vi "XML_Read_Modbus_Items.vi"(8 "error in (no error)":errorcluster, 11 ".NET Refnum in":refnum<k24>) -> (0 "error out":errorcluster, 2 "Array":T1[](array[typedef]), 3 ".NET Refnum out":refnum<k24>)   [LabVIEW 2014, in "XML_Deserializer.lvlib"]
uses:
  XML_Deserializer.lvlib
  C:/Users/vruault.AMER/Desktop/Source code/XML Deserializer/.NET Files/bin/Debug/Modbus_CD_XML_Deserializer.dll
  .NET Files/bin/Debug/Modbus_CD_XML_Deserializer.dll
  Controls/Modbus_Items.ctl
  Controls/Modbus_Item_Type.ctl
  Shared/Modbus Shared.lvlib
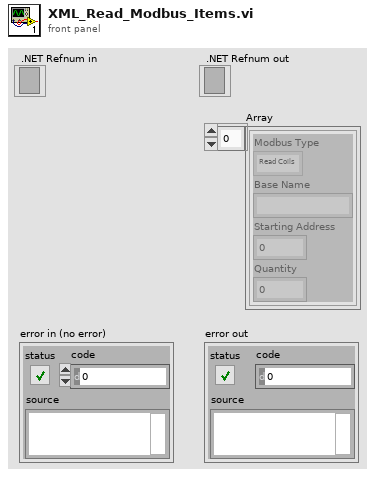
[diagram p1: front panel]
types:
  T1 = typedef "Modbus Shared.lvlib/Modbus_Items.ctl" = cluster{"Modbus Type":T2, "Base Name":string, "Starting Address":u16, "Quantity":u16}
  T2 = typedef "Modbus Shared.lvlib/Modbus_Item_Type.ctl" = enum16{"Read Coils", "Read Discrete Inputs", "Read Holding Registers", "Read Input Registers", "Write Multiple Coils", "Write Multiple Holding Registers", "Write Single Coil", "Write Single Holding Register", "Write Multiple Discrete Inputs", "Write Multiple Input Registers"}
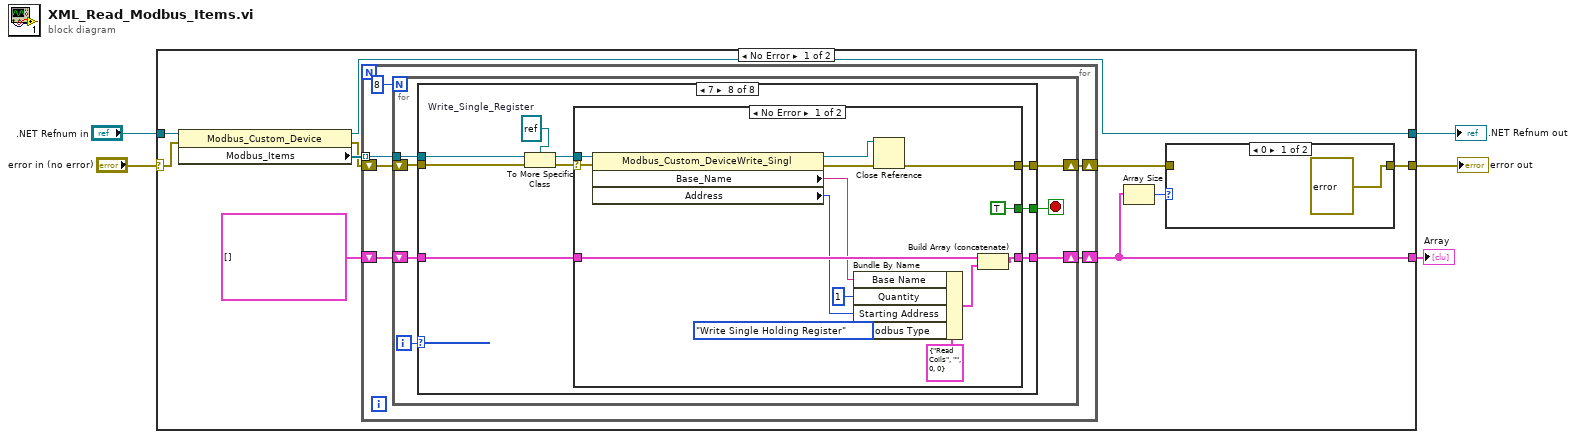
[diagram p0: block diagram]
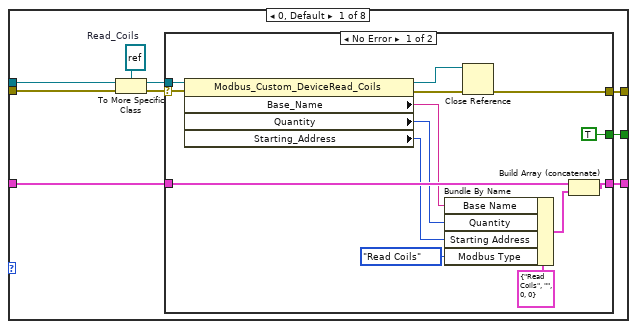
[diagram p3: hidden frame]
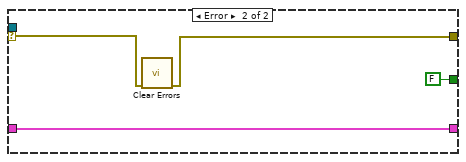
[diagram p4: hidden frame]
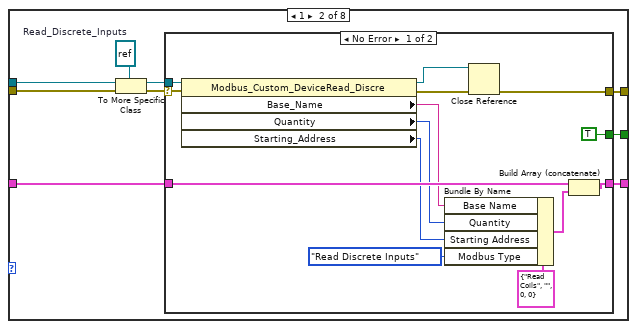
[diagram p5: hidden frame]
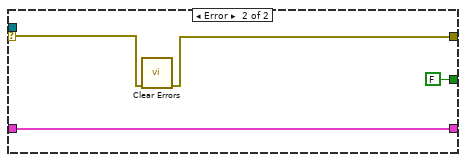
[diagram p6: hidden frame]
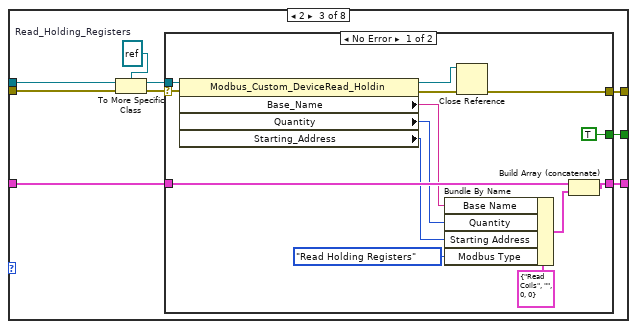
[diagram p7: hidden frame]
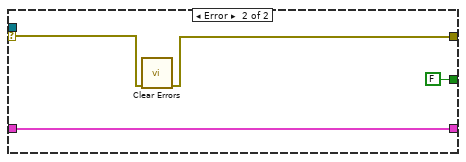
[diagram p8: hidden frame]
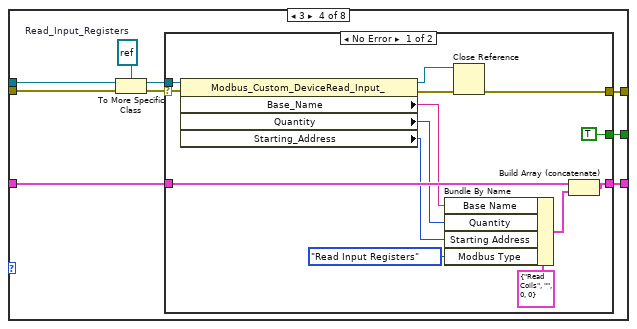
[diagram p9: hidden frame]
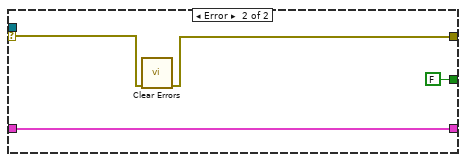
[diagram p10: hidden frame]
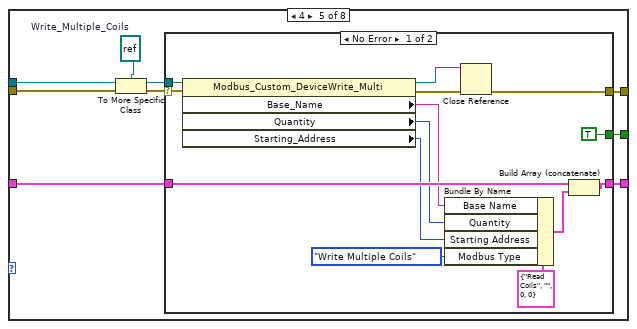
[diagram p11: hidden frame]
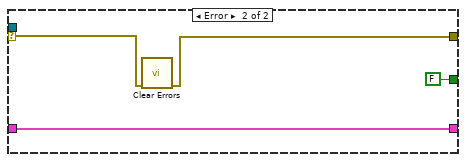
[diagram p12: hidden frame]
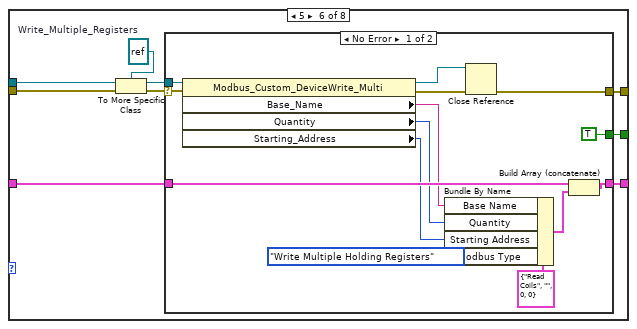
[diagram p13: hidden frame]
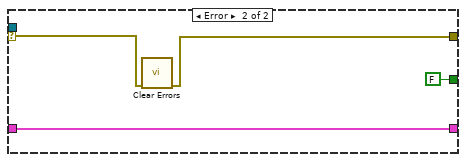
[diagram p14: hidden frame]
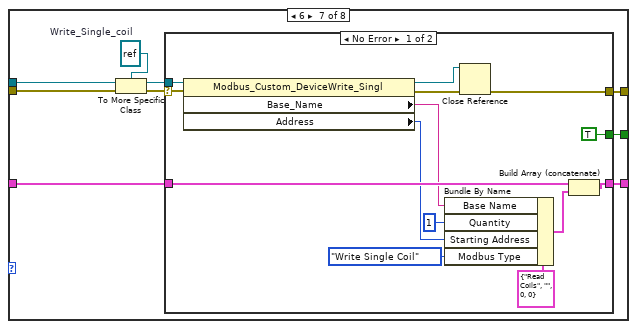
[diagram p15: hidden frame]
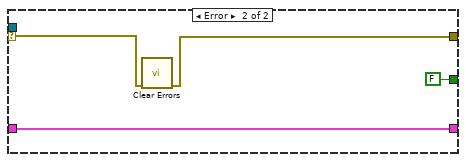
[diagram p16: hidden frame]
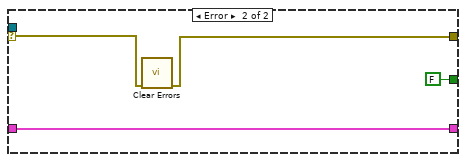
[diagram p17: hidden frame]
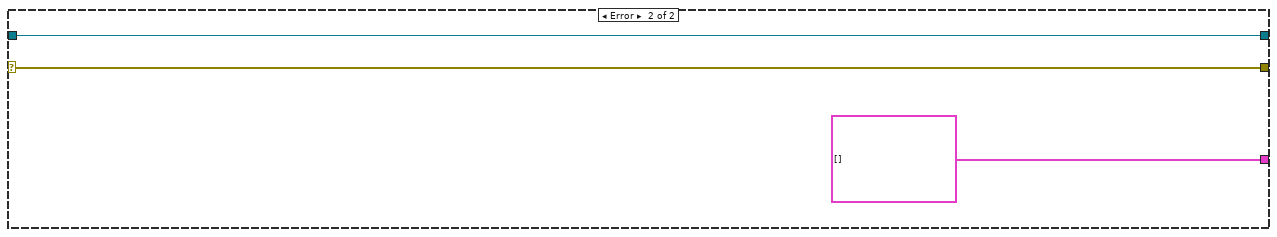
[diagram p18: hidden frame]
diagram:
  n1 = case shown="No Error" "error in (no error)" {
    selector: "error in (no error)" -> [w11 w249]
    tunnel: [w9 T1[] []] -> w1
    tunnel: [w6 w249] -> w2
    tunnel: ".NET Refnum in" -> [w12 w247]
    tunnel: [w10 w247] -> w5
    frame No Error {
      n2 = property class="Modbus_Custom_Device"(reference=w12, error in=w11) -> (reference out=w10:refnum<k24>, error out=w13:errorcluster, "Modbus_Items"=w15:refnum<k24>[])
      n3 = for {
        tunnel: w15 -> [w23] mode=indexing
        shift-right: [w21] -> w9
        shift-left: T1[] [] -> [w22]
        shift-right: [w20] -> w7
        shift-left: w13 -> [w19]
        n4 = for {
          N: 8 -> [_]
          tunnel: w23 -> [w30]
          shift-right: [w26] -> w21
          shift-left: w22 -> [w27]
          shift-right: [w25] -> w20
          shift-left: w19 -> [w29]
          i -> [w28]
          stop <- w24 stop-if-true
          n5 = case shown="7" w28 {
            tunnel: w30 -> [w39 w66 w93 w120 w147 w174 w201 w228]
            tunnel: w29 -> [w38 w65 w92 w119 w146 w173 w200 w227]
            tunnel: w27 -> [w34 w62 w89 w116 w143 w170 w197 w224]
            tunnel: [w33 w61 w88 w115 w142 w169 w196 w223] -> w26
            tunnel: [w32 w60 w87 w114 w141 w168 w195 w222] -> w25
            tunnel: [w31 w59 w86 w113 w140 w167 w194 w221] -> w24
            frame 0, Default {
              w37 = refnum<k24> refnum  # Read_Coils
              n6 = To More Specific Class(target class=w37, reference=w39, error in=w38) -> (specific class reference=w36:refnum<k24>, error out=w35:errorcluster)
              n7 = case shown="No Error" w35 {
                selector: w35 -> [w52 w57]
                tunnel: w36 -> [w53 _]
                tunnel: w34 -> [w50 w54]
                tunnel: [w49 w54] -> w33
                tunnel: [w41 w55] -> w32
                tunnel: [TRUE FALSE] -> w31
                frame No Error {
                  n8 = property class="Modbus_Custom_DeviceRead_Coils"(reference=w53, error in=w52) -> (reference out=w40:refnum<k24>, error out=w42:errorcluster, "Base_Name"=w45:string, "Quantity"=w44:u16, "Starting_Address"=w43:u16)
                  n9 = Bundle By Name(cluster=T1 {"Modbus Type"=enum."Read Coils", "Base Name"="", "Starting Address"=0, "Quantity"=0} ("Modbus Items"), "Base Name"=w45, "Quantity"=w44, "Starting Address"=w43, "Modbus Type"=Modbus_Item_Type."Read Coils") -> (w48:T1)
                  n10 = Close Reference(reference=w40, error in (no error)=w42) -> (error out=w41:errorcluster)
                  n11 = Build Array (concatenate)(w50, w48) -> (w49:T1[])
                }
                frame Error {
                  n12 = call <vilib>:"Clear Errors.vi"("error in (no error)"=w57) -> ("error out"=w55:errorcluster)  [unwired: 5 in, 1 out]
                }
              }
            }
            frame 1 {
              w58 = refnum<k24> refnum  # Read_Discrete_Inputs
              n13 = To More Specific Class(target class=w58, reference=w66, error in=w65) -> (specific class reference=w64:refnum<k24>, error out=w63:errorcluster)
              n14 = case shown="No Error" w63 {
                selector: w63 -> [w79 w84]
                tunnel: w64 -> [w80 _]
                tunnel: w62 -> [w77 w81]
                tunnel: [w76 w81] -> w61
                tunnel: [w67 w82] -> w60
                tunnel: [TRUE FALSE] -> w59
                frame No Error {
                  n15 = property class="Modbus_Custom_DeviceRead_Discre"(reference=w80, error in=w79) -> (reference out=w69:refnum<k24>, error out=w68:errorcluster, "Base_Name"=w72:string, "Quantity"=w71:u16, "Starting_Address"=w70:u16)
                  n16 = Bundle By Name(cluster=T1 {"Modbus Type"=enum."Read Coils", "Base Name"="", "Starting Address"=0, "Quantity"=0} ("Modbus Items"), "Base Name"=w72, "Quantity"=w71, "Starting Address"=w70, "Modbus Type"=Modbus_Item_Type."Read Discrete Inputs") -> (w75:T1)
                  n17 = Close Reference(reference=w69, error in (no error)=w68) -> (error out=w67:errorcluster)
                  n18 = Build Array (concatenate)(w77, w75) -> (w76:T1[])
                }
                frame Error {
                  n19 = call <vilib>:"Clear Errors.vi"("error in (no error)"=w84) -> ("error out"=w82:errorcluster)  [unwired: 5 in, 1 out]
                }
              }
            }
            frame 2 {
              w85 = refnum<k24> refnum  # Read_Holding_Registers
              n20 = To More Specific Class(target class=w85, reference=w93, error in=w92) -> (specific class reference=w91:refnum<k24>, error out=w90:errorcluster)
              n21 = case shown="No Error" w90 {
                selector: w90 -> [w106 w111]
                tunnel: w91 -> [w107 _]
                tunnel: w89 -> [w104 w108]
                tunnel: [w103 w108] -> w88
                tunnel: [w94 w109] -> w87
                tunnel: [TRUE FALSE] -> w86
                frame No Error {
                  n22 = property class="Modbus_Custom_DeviceRead_Holdin"(reference=w107, error in=w106) -> (reference out=w96:refnum<k24>, error out=w95:errorcluster, "Base_Name"=w99:string, "Quantity"=w98:u16, "Starting_Address"=w97:u16)
                  n23 = Bundle By Name(cluster=T1 {"Modbus Type"=enum."Read Coils", "Base Name"="", "Starting Address"=0, "Quantity"=0} ("Modbus Items"), "Base Name"=w99, "Quantity"=w98, "Starting Address"=w97, "Modbus Type"=Modbus_Item_Type."Read Holding Registers") -> (w102:T1)
                  n24 = Close Reference(reference=w96, error in (no error)=w95) -> (error out=w94:errorcluster)
                  n25 = Build Array (concatenate)(w104, w102) -> (w103:T1[])
                }
                frame Error {
                  n26 = call <vilib>:"Clear Errors.vi"("error in (no error)"=w111) -> ("error out"=w109:errorcluster)  [unwired: 5 in, 1 out]
                }
              }
            }
            frame 3 {
              w112 = refnum<k24> refnum  # Read_Input_Registers
              n27 = To More Specific Class(target class=w112, reference=w120, error in=w119) -> (specific class reference=w118:refnum<k24>, error out=w117:errorcluster)
              n28 = case shown="No Error" w117 {
                selector: w117 -> [w133 w138]
                tunnel: w118 -> [w134 _]
                tunnel: w116 -> [w131 w135]
                tunnel: [w130 w135] -> w115
                tunnel: [w121 w136] -> w114
                tunnel: [TRUE FALSE] -> w113
                frame No Error {
                  n29 = property class="Modbus_Custom_DeviceRead_Input_"(reference=w134, error in=w133) -> (reference out=w123:refnum<k24>, error out=w122:errorcluster, "Base_Name"=w126:string, "Quantity"=w125:u16, "Starting_Address"=w124:u16)
                  n30 = Bundle By Name(cluster=T1 {"Modbus Type"=enum."Read Coils", "Base Name"="", "Starting Address"=0, "Quantity"=0} ("Modbus Items"), "Base Name"=w126, "Quantity"=w125, "Starting Address"=w124, "Modbus Type"=Modbus_Item_Type."Read Input Registers") -> (w129:T1)
                  n31 = Close Reference(reference=w123, error in (no error)=w122) -> (error out=w121:errorcluster)
                  n32 = Build Array (concatenate)(w131, w129) -> (w130:T1[])
                }
                frame Error {
                  n33 = call <vilib>:"Clear Errors.vi"("error in (no error)"=w138) -> ("error out"=w136:errorcluster)  [unwired: 5 in, 1 out]
                }
              }
            }
            frame 4 {
              w139 = refnum<k24> refnum  # Write_Multiple_Coils
              n34 = To More Specific Class(target class=w139, reference=w147, error in=w146) -> (specific class reference=w145:refnum<k24>, error out=w144:errorcluster)
              n35 = case shown="No Error" w144 {
                selector: w144 -> [w160 w165]
                tunnel: w145 -> [w161 _]
                tunnel: w143 -> [w158 w162]
                tunnel: [w157 w162] -> w142
                tunnel: [w149 w163] -> w141
                tunnel: [TRUE FALSE] -> w140
                frame No Error {
                  n36 = property class="Modbus_Custom_DeviceWrite_Multi"(reference=w161, error in=w160) -> (reference out=w148:refnum<k24>, error out=w150:errorcluster, "Base_Name"=w153:string, "Quantity"=w152:u16, "Starting_Address"=w151:u16)
                  n37 = Bundle By Name(cluster=T1 {"Modbus Type"=enum."Read Coils", "Base Name"="", "Starting Address"=0, "Quantity"=0} ("Modbus Items"), "Base Name"=w153, "Quantity"=w152, "Starting Address"=w151, "Modbus Type"=Modbus_Item_Type."Write Multiple Coils") -> (w156:T1)
                  n38 = Close Reference(reference=w148, error in (no error)=w150) -> (error out=w149:errorcluster)
                  n39 = Build Array (concatenate)(w158, w156) -> (w157:T1[])
                }
                frame Error {
                  n40 = call <vilib>:"Clear Errors.vi"("error in (no error)"=w165) -> ("error out"=w163:errorcluster)  [unwired: 5 in, 1 out]
                }
              }
            }
            frame 5 {
              w166 = refnum<k24> refnum  # Write_Multiple_Registers
              n41 = To More Specific Class(target class=w166, reference=w174, error in=w173) -> (specific class reference=w172:refnum<k24>, error out=w171:errorcluster)
              n42 = case shown="No Error" w171 {
                selector: w171 -> [w187 w192]
                tunnel: w172 -> [w188 _]
                tunnel: w170 -> [w185 w189]
                tunnel: [w184 w189] -> w169
                tunnel: [w175 w190] -> w168
                tunnel: [TRUE FALSE] -> w167
                frame No Error {
                  n43 = property class="Modbus_Custom_DeviceWrite_Multi"(reference=w188, error in=w187) -> (reference out=w176:refnum<k24>, error out=w177:errorcluster, "Base_Name"=w180:string, "Quantity"=w179:u16, "Starting_Address"=w178:u16)
                  n44 = Bundle By Name(cluster=T1 {"Modbus Type"=enum."Read Coils", "Base Name"="", "Starting Address"=0, "Quantity"=0} ("Modbus Items"), "Base Name"=w180, "Quantity"=w179, "Starting Address"=w178, "Modbus Type"=Modbus_Item_Type."Write Multiple Holding Registers") -> (w183:T1)
                  n45 = Close Reference(reference=w176, error in (no error)=w177) -> (error out=w175:errorcluster)
                  n46 = Build Array (concatenate)(w185, w183) -> (w184:T1[])
                }
                frame Error {
                  n47 = call <vilib>:"Clear Errors.vi"("error in (no error)"=w192) -> ("error out"=w190:errorcluster)  [unwired: 5 in, 1 out]
                }
              }
            }
            frame 6 {
              w193 = refnum<k24> refnum  # Write_Single_coil
              n48 = To More Specific Class(target class=w193, reference=w201, error in=w200) -> (specific class reference=w199:refnum<k24>, error out=w198:errorcluster)
              n49 = case shown="No Error" w198 {
                selector: w198 -> [w214 w219]
                tunnel: w199 -> [w215 _]
                tunnel: w197 -> [w212 w216]
                tunnel: [w211 w216] -> w196
                tunnel: [w202 w217] -> w195
                tunnel: [TRUE FALSE] -> w194
                frame No Error {
                  n50 = property class="Modbus_Custom_DeviceWrite_Singl"(reference=w215, error in=w214) -> (reference out=w204:refnum<k24>, error out=w203:errorcluster, "Base_Name"=w207:string, "Address"=w206:u16)
                  n51 = Bundle By Name(cluster=T1 {"Modbus Type"=enum."Read Coils", "Base Name"="", "Starting Address"=0, "Quantity"=0} ("Modbus Items"), "Base Name"=w207, "Quantity"=u16 1, "Starting Address"=w206, "Modbus Type"=Modbus_Item_Type."Write Single Coil") -> (w210:T1)
                  n52 = Close Reference(reference=w204, error in (no error)=w203) -> (error out=w202:errorcluster)
                  n53 = Build Array (concatenate)(w212, w210) -> (w211:T1[])
                }
                frame Error {
                  n54 = call <vilib>:"Clear Errors.vi"("error in (no error)"=w219) -> ("error out"=w217:errorcluster)  [unwired: 5 in, 1 out]
                }
              }
            }
            frame 7 {
              w220 = refnum<k24> refnum  # Write_Single_Register
              n55 = To More Specific Class(target class=w220, reference=w228, error in=w227) -> (specific class reference=w226:refnum<k24>, error out=w225:errorcluster)
              n56 = case shown="No Error" w225 {
                selector: w225 -> [w241 w246]
                tunnel: w226 -> [w242 _]
                tunnel: w224 -> [w239 w243]
                tunnel: [w238 w243] -> w223
                tunnel: [w229 w244] -> w222
                tunnel: [TRUE FALSE] -> w221
                frame No Error {
                  n57 = property class="Modbus_Custom_DeviceWrite_Singl"(reference=w242, error in=w241) -> (reference out=w231:refnum<k24>, error out=w230:errorcluster, "Base_Name"=w234:string, "Address"=w233:u16)
                  n58 = Bundle By Name(cluster=T1 {"Modbus Type"=enum."Read Coils", "Base Name"="", "Starting Address"=0, "Quantity"=0} ("Modbus Items"), "Base Name"=w234, "Quantity"=u16 1, "Starting Address"=w233, "Modbus Type"=Modbus_Item_Type."Write Single Holding Register") -> (w237:T1)
                  n59 = Close Reference(reference=w231, error in (no error)=w230) -> (error out=w229:errorcluster)
                  n60 = Build Array (concatenate)(w239, w237) -> (w238:T1[])
                }
                frame Error {
                  n61 = call <vilib>:"Clear Errors.vi"("error in (no error)"=w246) -> ("error out"=w244:errorcluster)  [unwired: 5 in, 1 out]
                }
              }
            }
          }
        }
      }
      n62 = Array Size(array=w9) -> (size(s)=w8:i32)
      n63 = case shown="0" w8 {
        tunnel: w7 -> [_ w17]
        tunnel: [errorcluster {"status"=TRUE, "code"=5003, "source"="Error in XML File: \"Modbus_Items\" tag doesn't have elements inside. At least one element is required."} ("error out") w17] -> w6
        frame 0 {
        }
        frame 1, Default {
        }
      }
    }
    frame Error {
    }
  }
  ".NET Refnum out" <- w5
  "error out" <- w2
  "Array" <- w1
